vi "Joystick Curve.vi"(2 "Right Axis Value":dbl, 3 "Left Axis Value":dbl) -> (0 "Modified Right Axis Value":dbl, 1 "Modified Left Axis Value":dbl)   [LabVIEW 2012]
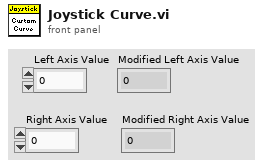
[diagram p1: front panel]
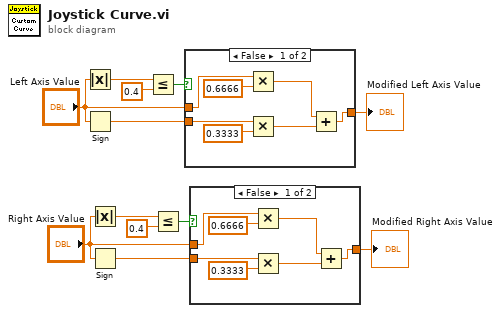
[diagram p0: block diagram]
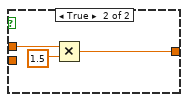
[diagram p2: hidden frame]
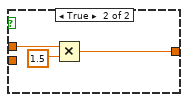
[diagram p3: hidden frame]
diagram:
  n1 = Absolute Value(x="Left Axis Value") -> (abs(x)=w8:dbl)
  n2 = Sign(1:"Left Axis Value") -> (0:w12:dbl)
  n3 = Absolute Value(x="Right Axis Value") -> (abs(x)=w2:dbl)
  n4 = Sign(1:"Right Axis Value") -> (0:w6:dbl)
  n5 = Less Or Equal?(x=w8, y=0.4) -> (x <= y?=w9:bool)
  n6 = Less Or Equal?(x=w2, y=0.4) -> (x <= y?=w3:bool)
  n7 = case shown="False" w9 {
    tunnel: "Left Axis Value" -> [w19 w21]
    tunnel: [w17 w20] -> w10
    tunnel: w12 -> [w15 _]
    frame False {
      n8 = Multiply(x=w19, y=0.6666) -> (x*y=w18:dbl)
      n9 = Multiply(x=w15, y=0.3333) -> (x*y=w16:dbl)
      n10 = Add(x=w18, y=w16) -> (x+y=w17:dbl)
    }
    frame True {
      n11 = Multiply(x=w21, y=1.5) -> (x*y=w20:dbl)
    }
  }
  "Modified Left Axis Value" <- w10
  n12 = case shown="False" w3 {
    tunnel: "Right Axis Value" -> [w29 w31]
    tunnel: [w27 w30] -> w4
    tunnel: w6 -> [w25 _]
    frame False {
      n13 = Multiply(x=w29, y=0.6666) -> (x*y=w28:dbl)
      n14 = Multiply(x=w25, y=0.3333) -> (x*y=w26:dbl)
      n15 = Add(x=w28, y=w26) -> (x+y=w27:dbl)
    }
    frame True {
      n16 = Multiply(x=w31, y=1.5) -> (x*y=w30:dbl)
    }
  }
  "Modified Right Axis Value" <- w4
